vi "ciclos6.vi"() -> ()   [LabVIEW 2013]
panel:
  in  "enceder":bool
  out "Rango3 151-220":bool
  out "Rango2 101-150":bool
  out "Rango1-100":bool
  out "Rango 151-220":dbl
  out "Rango 101-150":dbl
  out "Rango 1-100":dbl
  out "velocidad":i32(knob) scale=0.0..220.0
  # "se tiene que contar cuantas veces la velocidad se genera en cada una de los\nrangos y se enciende el led que corresponde a cada uno de los rangos.\nhacerlo hasta apagar el auto"
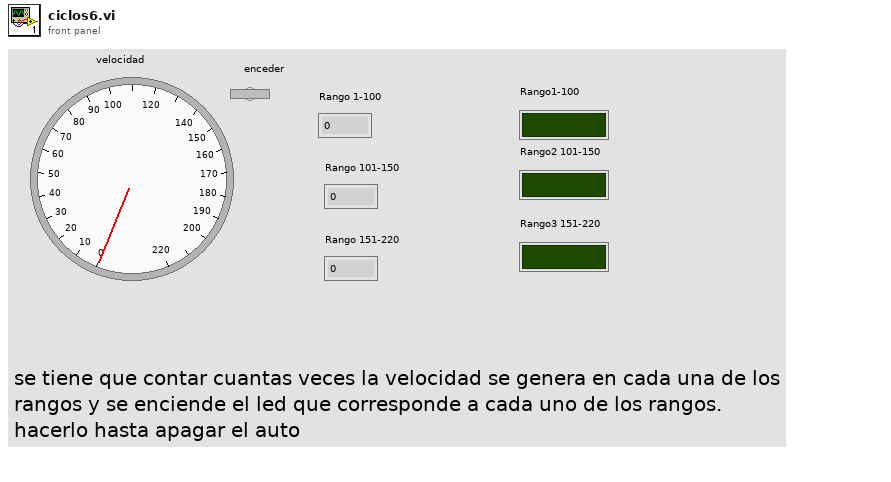
[diagram p1: front panel]
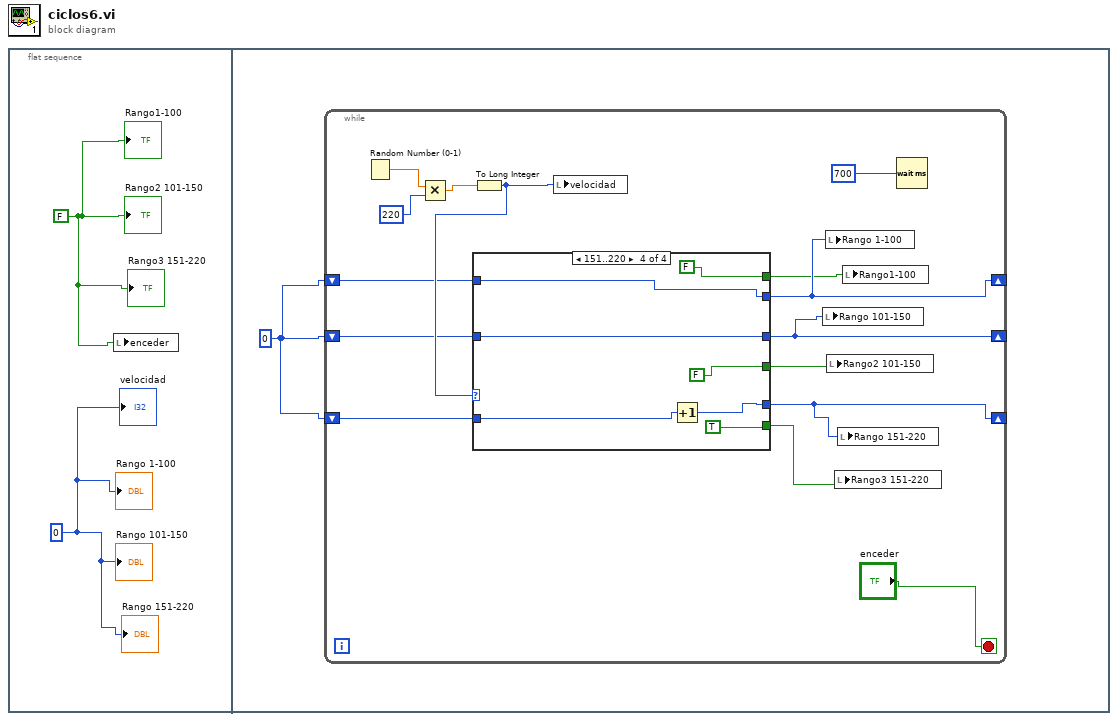
[diagram p0: block diagram]
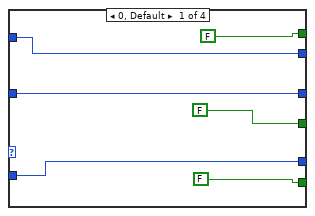
[diagram p2: hidden frame]
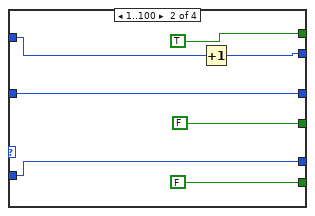
[diagram p3: hidden frame]
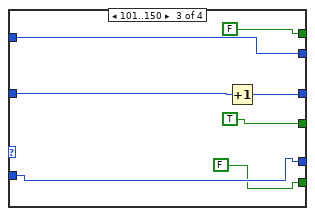
[diagram p4: hidden frame]
diagram:
  n1 = flat-sequence {
    frame #0 {
      w1 = FALSE
      w2 = 0
      n2 = local write "enceder"(w1) -> ()
      "velocidad" <- w2
      "Rango1-100" <- w1
      "Rango2 101-150" <- w1
      "Rango3 151-220" <- w1
      "Rango 1-100" <- w2
      "Rango 101-150" <- w2
      "Rango 151-220" <- w2
    }
    frame #1 {
      w3 = 0
      n3 = while {
        shift-right: [w10] -> _
        shift-left: w3 -> [w13]
        shift-right: [w8] -> _
        shift-left: w3 -> [w12]
        shift-right: [w6] -> _
        shift-left: w3 -> [w11]
        stop <- "enceder" stop-if-true
        n4 = Random Number (0-1)() -> (number: 0 to 1=w17:dbl)
        n5 = Multiply(x=w17, y=220) -> (x*y=w15:dbl)
        n6 = To Long Integer(number=w15) -> (32bit integer=w14:i32)
        n7 = case shown="151..220" w14 {
          tunnel: [w24 w29 w38 w45] -> w10
          tunnel: w13 -> [w24 w28 w38 w45]
          tunnel: [w23 w30 w37 w42] -> w8
          tunnel: w12 -> [w23 w30 w36 w42]
          tunnel: [w22 w31 w35 w40] -> w6
          tunnel: w11 -> [w22 w31 w35 w41]
          tunnel: [FALSE FALSE TRUE FALSE] -> w7
          tunnel: [FALSE FALSE FALSE TRUE] -> w5
          tunnel: [FALSE TRUE FALSE FALSE] -> w9
          frame 0, Default {
          }
          frame 1..100 {
            n8 = Increment(x=w28) -> (x+1=w29:i32)
          }
          frame 101..150 {
            n9 = Increment(x=w36) -> (x+1=w37:i32)
          }
          frame 151..220 {
            n10 = Increment(x=w41) -> (x+1=w40:i32)
          }
        }
        n11 = local write "velocidad"(w14) -> ()
        n12 = local write "Rango 101-150"(w8) -> ()
        n13 = local write "Rango 1-100"(w10) -> ()
        n14 = local write "Rango2 101-150"(w7) -> ()
        n15 = local write "Rango3 151-220"(w5) -> ()
        n16 = local write "Rango 151-220"(w6) -> ()
        n17 = local write "Rango1-100"(w9) -> ()
        n18 = Wait (ms)(milliseconds to wait=700) -> ()  [unwired: 1 out]
      }
    }
  }
